vi "merFISH_close.vi"(0 "queue DAQ":refnum<queue>, 1 "queue ASI stage":refnum<queue>, 2 "queue FPGA":refnum<queue>, 5 "queue CAMERA":refnum<queue>, 7 "queue pump":refnum<queue>, 9 "queue piezo":refnum<queue>, 11 "error in":errorcluster, 12 "Measure QPD":bool) -> (15 "error out":errorcluster)   [LabVIEW 2015]
uses:
  CONTROLS/Q_ASI_stage_element.ctl
  CONTROLS/Q_DAQ_element.ctl
  CONTROLS/Q_camera_element.ctl
  CONTROLS/Q_MCL_piezo_element.ctl
  CONTROLS/Q_PUMP_element.ctl
  CONTROLS/Q_FPGA_element.ctl
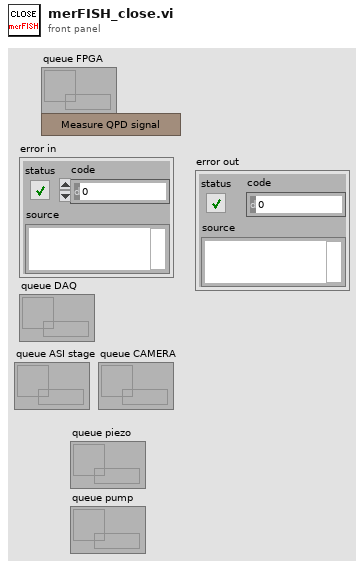
[diagram p1: front panel]
types:
  T1 = typedef "Q_FPGA_element.ctl" = cluster{"variant":variant, "Instruction":enum16{"FPGA_idle", "FPGA_initialize", "FPGA_error", "FPGA_security_stop", "FPGA_laser", "FPGA_start_stop_measure_QPD", "FPGA_measure_QPD", "FPGA_measure_QPD_noise", "FPGA_stop_measure_QPD", "FPGA_init_autofocus", "FPGA_init_single_scan", "FPGA_stop_single_scan", "FPGA_init_merFISH", "FPGA_measure_QPD_merFISH", "FPGA_init_scan_merFISH", "FPGA_scan_merFISH", "FPGA_close_merFISH", "FPGA_stop"}}
  T2 = typedef "Q_PUMP_element.ctl" = cluster{"variant":variant, "Instruction":enum16{"PUMP_idle", "PUMP_initialize", "PUMP_error", "PUMP_security_stop", "PUMP_read_pressure", "PUMP_change_pressure", "PUMP_init_merFISH", "PUMP_change_presure_merFISH", "PUMP_zero_pressure_merFISH", "PUMP_close_merFISH", "PUMP_stop"}}
  T3 = typedef "Q_MCL_piezo_element.ctl" = cluster{"variant":variant, "Instruction":enum16{"Piezo_idle", "Piezo_initialize", "Piezo_error", "Piezo_security_stop", "Piezo_read_z", "Piezo_move_z", "Piezo_keyboard_move", "Piezo_close_autofocus_calibration_ramp", "Piezo_change_init_state", "Piezo_init_autofocus", "Piezo_init_autofocus_merFISH_TL", "Piezo_autofocus", "Piezo_autofocus_merFISH_TL", "Piezo_stop_autofocus", "Piezo_stop_autofocus_merFISH_TL", "Piezo_autofocus_lost", "Piezo_resume_autofocus_merFISH_TL", "Piezo_check_z_position_merFISH_TL", "Piezo_init_ramp", "Piezo_move_z_ramp", "Piezo_close_ramp", "Piezo_close_merFISH", "Piezo_stop"}}
  T4 = typedef "Q_ASI_stage_element.ctl" = cluster{"variant":variant, "Instruction":enum16{"ASI_idle", "ASI_initialize", "ASI_error", "ASI_security_stop", "ASI_read_XYZ", "ASI_up", "ASI_down", "ASI_left", "ASI_right", "ASI_save_XY", "ASI_move_to_XY", "ASI_brightfield", "ASI_init_scan", "ASI_init_merFISH", "ASI_move_to_XY_merFISH", "ASI_move_to_Z_merFISH", "ASI_init_autofocus_search_merFISH", "ASI_close_autofocus_search_merFISH", "ASI_adjust_piezo_autofocus_merFISH", "ASI_set_piezo_autofocus_to_reference_position_merFISH_TL", "ASI_close_merFISH", "ASI_stop"}}
  T5 = typedef "Q_DAQ_element.ctl" = cluster{"variant":variant, "Instruction":enum16{"DAQ_idle", "DAQ_initialize", "DAQ_error", "DAQ_security_stop", "DAQ_init_single_scan", "DAQ_single_scan", "DAQ_init_merFISH", "DAQ_scan_merFISH", "DAQ_photobleaching_merFISH", "DAQ_close_merFISH", "DAQ_stop"}}
  T6 = typedef "Q_camera_element.ctl" = cluster{"variant":variant, "Instruction":enum16{"CAMERA_idle", "CAMERA_initialize", "CAMERA_error", "CAMERA_security_stop", "CAMERA_not_acquiring", "CAMERA_acquiring", "CAMERA_start_acquiring", "CAMERA_stop_acquiring", "CAMERA_change_exposure", "CAMERA_define_ROI", "CAMERA_cooler", "CAMERA_acquire_movie", "CAMERA_init_scan", "CAMERA_check_image_scan", "CAMERA_close_scan", "CAMERA_init_merFISH", "CAMERA_start_acquiring_merFISH", "CAMERA_close_scan_merFISH", "CAMERA_close_merFISH", "CAMERA_STOP"}}
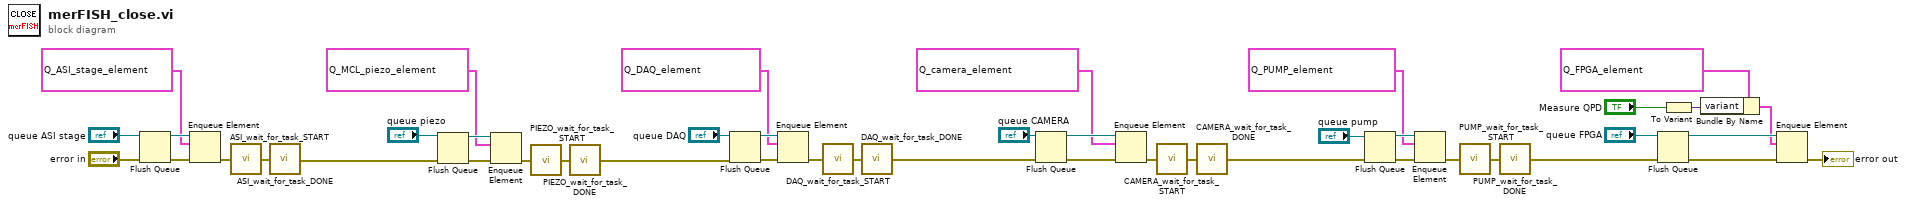
[diagram p0: block diagram]
diagram:
  n1 = Flush Queue(queue="queue ASI stage", error in (no error)="error in") -> (queue out=w30:refnum<queue>, error out=w31:errorcluster)  [unwired: 1 out]
  n2 = Enqueue Element(queue=w30, element=T4 {"variant"=variant, "Instruction"=enum."ASI_close_merFISH"} ("Q_ASI_stage"), error in (no error)=w31) -> (error out=w29:errorcluster)  [unwired: 1 in, 2 out]
  n3 = call "ASI_wait_for_task_START.vi"("error in"=w29) -> ("error out"=w28:errorcluster)
  n4 = call "ASI_wait_for_task_DONE.vi"("error in"=w28) -> ("error out"=w25:errorcluster)
  n5 = Flush Queue(queue="queue piezo", error in (no error)=w25) -> (queue out=w22:refnum<queue>, error out=w24:errorcluster)  [unwired: 1 out]
  n6 = Enqueue Element(queue=w22, element=T3 {"variant"=variant, "Instruction"=enum."Piezo_close_merFISH"}, error in (no error)=w24) -> (error out=w23:errorcluster)  [unwired: 1 in, 2 out]
  n7 = call "PIEZO_wait_for_task_START.vi"("error in"=w23) -> ("error out"=w20:errorcluster)
  n8 = call "PIEZO_wait_for_task_DONE.vi"("error in"=w20) -> ("error out"=w19:errorcluster)
  n9 = Flush Queue(queue="queue DAQ", error in (no error)=w19) -> (queue out=w35:refnum<queue>, error out=w34:errorcluster)  [unwired: 1 out]
  n10 = Enqueue Element(queue=w35, element=T5 {"variant"=variant, "Instruction"=enum."DAQ_close_merFISH"} ("Q_DAQ"), error in (no error)=w34) -> (error out=w7:errorcluster)  [unwired: 1 in, 2 out]
  n11 = call "DAQ_wait_for_task_START.vi"("error in"=w7) -> ("error out"=w36:errorcluster)
  n12 = call "DAQ_wait_for_task_DONE.vi"("error in"=w36) -> ("error out"=w33:errorcluster)
  n13 = Flush Queue(queue="queue CAMERA", error in (no error)=w33) -> (queue out=w40:refnum<queue>, error out=w39:errorcluster)  [unwired: 1 out]
  n14 = Enqueue Element(queue=w40, element=T6 {"variant"=variant, "Instruction"=enum."CAMERA_close_merFISH"} ("Q_ANDOR_element"), error in (no error)=w39) -> (error out=w41:errorcluster)  [unwired: 1 in, 2 out]
  n15 = call "CAMERA_wait_for_task_START.vi"("error in"=w41) -> ("error out"=w42:errorcluster)
  n16 = call "CAMERA_wait_for_task_DONE.vi"("error in"=w42) -> ("error out"=w18:errorcluster)
  n17 = Flush Queue(queue="queue pump", error in (no error)=w18) -> (queue out=w15:refnum<queue>, error out=w16:errorcluster)  [unwired: 1 out]
  n18 = Enqueue Element(queue=w15, element=T2 {"variant"=variant, "Instruction"=enum."PUMP_close_merFISH"}, error in (no error)=w16) -> (error out=w13:errorcluster)  [unwired: 1 in, 2 out]
  n19 = call "PUMP_wait_for_task_START.vi"("error in"=w13) -> ("error out"=w12:errorcluster)
  n20 = call "PUMP_wait_for_task_DONE.vi"("error in"=w12) -> ("error out"=w6:errorcluster)
  n21 = Flush Queue(queue="queue FPGA", error in (no error)=w6) -> (queue out=w8:refnum<queue>, error out=w10:errorcluster)  [unwired: 1 out]
  n22 = To Variant(anything="Measure QPD") -> (Variant=w2:variant)
  n23 = Bundle By Name(cluster=T1 {"variant"=variant, "Instruction"=enum."FPGA_close_merFISH"} ("element"), "variant"=w2) -> (w3:T1)
  n24 = Enqueue Element(queue=w8, element=w3, error in (no error)=w10) -> (error out=→"error out":errorcluster)  [unwired: 1 in, 2 out]
